vi "VisionGetCameraConnectStatus.vi"() -> (0 "Vision Conn FrontRight":bool, 1 "Vision Conn RearBack":bool, 2 "Vision Conn RearRight":bool, 3 "Vision Conn FrontLeft":bool)   [LabVIEW 2023]
uses:
  VisionGlobal.vi
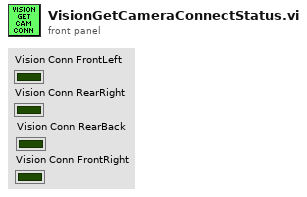
[diagram p1: front panel]
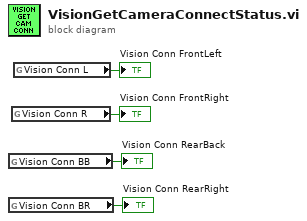
[diagram p0: block diagram]
diagram:
  n1 = global read "VisionGlobal.vi" "Vision Conn BB"() -> (→"Vision Conn RearBack":bool)
  n2 = global read "VisionGlobal.vi" "Vision Conn BR"() -> (→"Vision Conn RearRight":bool)
  n3 = global read "VisionGlobal.vi" "Vision Conn R"() -> (→"Vision Conn FrontRight":bool)
  n4 = global read "VisionGlobal.vi" "Vision Conn L"() -> (→"Vision Conn FrontLeft":bool)
